vi "Data.OnCompile.Execute.vi"(8 "error in":errorcluster, 10 "VS Ref Groups":T2(array[cluster]) {"VS Refs" format="%.0x"}, 11 "Custom Device Ref":T1 format="%.0x") -> (0 "error out":errorcluster, 3 "Custom Device Ref":T1 format="%.0x")   [LabVIEW 2023, in "Data Access System Explorer.lvlib"]
uses:
  Data Access System Explorer.lvlib
  <vilib>/NI VeriStand/Custom Device API/Custom Device API.lvlib
  <vilib>/NI VeriStand/Custom Device API/Data Reference.ctl
  <vilib>/NI VeriStand/Custom Device API/Block Data Reference.ctl
  <vilib>/NI VeriStand/Custom Device API/Set Item Property (Variant).vi
  <vilib>/NI VeriStand/Custom Device API/Data Access Type.ctl
  <vilib>/NI VeriStand/Custom Device API/Custom Device Item Ref.ctl
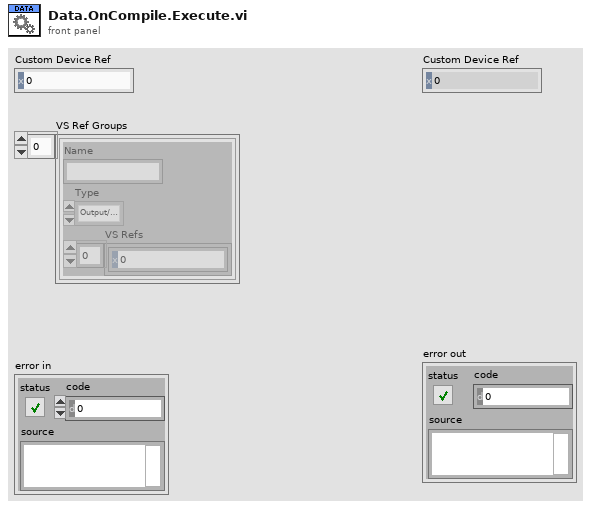
[diagram p1: front panel]
types:
  T1 = typedef "Custom Device API.lvlib/Custom Device Item Ref.ctl" = u64
  T2 = cluster{"Name":string, "Type":enum16{"Output/Write", "Input/Read", "Input/ReadWrite"}, "VS Refs":T1[]}[]
  T3 = typedef "Custom Device API.lvlib/Block Data Reference.ctl" = cluster{"Data Reference":T4, "Offset":u64, "Length":u64}
  T4 = typedef "Custom Device API.lvlib/Data Reference.ctl" = i32
  T5 = cluster{"Refs":T4[], "Values":dbl[], "Reset Values":dbl[]}[]
  T6 = cluster{"Read":cluster{"Refs":T3[], "Values":dbl[]}[], "Write":cluster{"Refs":T3[], "Values":dbl[]}[], "ReadWrite":cluster{"Refs":T4[], "Values":dbl[], "Reset Values":dbl[]}[], "LUT":variant}
  T7 = typedef "Custom Device API.lvlib/Data Access Type.ctl" = enum16{"Read", "Write"}
  T8 = cluster{"Refs":T4[], "Values":dbl[], "Reset Values":dbl[]}
  T9 = enum16{"Output/Write", "Input/Read", "Input/ReadWrite"}
  T10 = typedef "Custom Device API.lvlib/Custom Device Channel.ctl" = cluster{"Type":T11, "Units":string, "Default Value":dbl, "Faultable":bool, "Scalable":bool}
  T11 = typedef "Custom Device API.lvlib/Custom Device Channel Type.ctl" = enum16{"Input", "Output"}
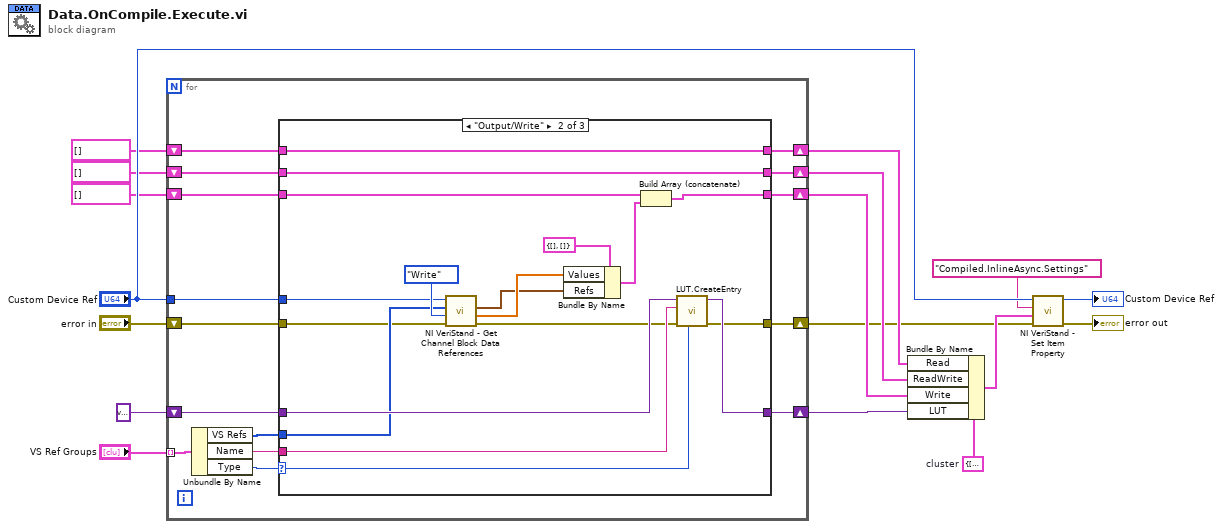
[diagram p0: block diagram]
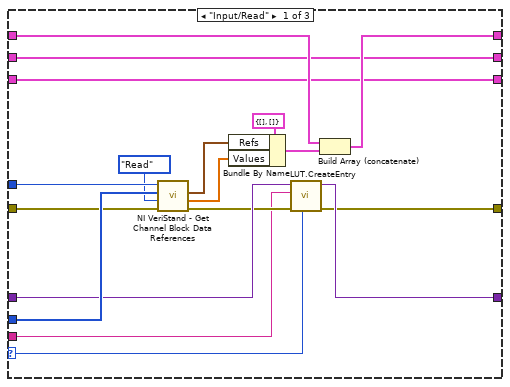
[diagram p2: hidden frame]
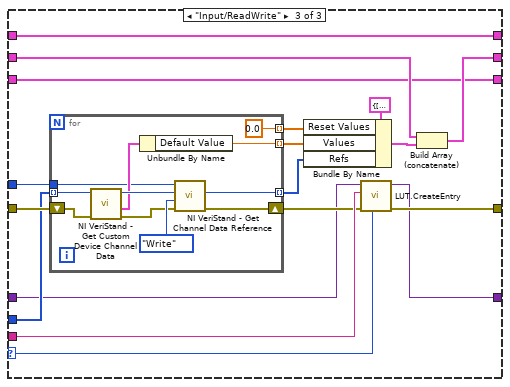
[diagram p3: hidden frame]
diagram:
  w13 = T6 {"Read"=[], "Write"=[], "ReadWrite"=[], "LUT"=variant}  # cluster
  n1 = for {
    tunnel: "VS Ref Groups" -> [w32] mode=indexing
    shift-right: [w30] -> w1
    shift-left: "error in" -> [w31]
    tunnel: "Custom Device Ref" -> [w28]
    shift-right: [w26] -> w2
    shift-left: variant ("LUT") -> [w27]
    shift-right: [w25] -> w4
    shift-left: cluster{"Refs":T3[], "Values":dbl[]}[] [] -> [w20]
    shift-right: [w22] -> w3
    shift-left: T5 [] -> [w21]
    shift-right: [w19] -> w5
    shift-left: cluster{"Refs":T3[], "Values":dbl[]}[] [] -> [w18]
    n2 = Unbundle By Name(w32) -> ("VS Refs"=w29:T1[], "Name"=w24:string, "Type"=w23:T9)
    n3 = case shown="\"Output/Write\"" w23 {
      selector: w23 -> [w38 w64 w79]
      tunnel: w31 -> [w47 w54 w83]
      tunnel: [w45 w65 w77] -> w30
      tunnel: w29 -> [w50 w56 w81]
      tunnel: w28 -> [w49 w57 w74]
      tunnel: w27 -> [w48 w67 w76]
      tunnel: [w46 w66 w75] -> w26
      tunnel: [w35 w62 w69] -> w25
      tunnel: w24 -> [w39 w68 w80]
      tunnel: [w34 w63 w71] -> w22
      tunnel: w21 -> [w34 w63 w73]
      tunnel: w20 -> [w37 w62 w69]
      tunnel: [w33 w60 w70] -> w19
      tunnel: w18 -> [w33 w59 w70]
      frame "Input/Read" {
        n4 = call <vilib>:"NI VeriStand - Get Channel Block Data References.vi"("error in (no error)"=w47, "Access"=Data_Access_Type."Read", "Channel Refs"=w50, "Device Ref in"=w49) -> ("error out"=w41:errorcluster, "Values Array"=w42:dbl[], "Block Data Refs"=w43:T3[])  [unwired: 4 in, 1 out]
        n5 = Bundle By Name(cluster=cluster{"Refs":T3[], "Values":dbl[]} {"Refs"=[], "Values"=[]}, "Refs"=w43, "Values"=w42) -> (w36:cluster{"Refs":T3[], "Values":dbl[]})
        n6 = call "LUT.CreateEntry.vi"("Type"=w38, "error in (no error)"=w41, "Name"=w39, "LUT"=w48) -> ("error out"=w45:errorcluster, "LUT"=w46:variant)  [unwired: 6 in]
        n7 = Build Array (concatenate)(w37, w36) -> (w35:cluster{"Refs":T3[], "Values":dbl[]}[])
      }
      frame "Output/Write" {
        n8 = call <vilib>:"NI VeriStand - Get Channel Block Data References.vi"("error in (no error)"=w54, "Access"=Data_Access_Type."Write", "Channel Refs"=w56, "Device Ref in"=w57) -> ("error out"=w53:errorcluster, "Values Array"=w55:dbl[], "Block Data Refs"=w51:T3[])  [unwired: 4 in, 1 out]
        n9 = Bundle By Name(cluster=cluster{"Refs":T3[], "Values":dbl[]} {"Refs"=[], "Values"=[]}, "Values"=w55, "Refs"=w51) -> (w61:cluster{"Refs":T3[], "Values":dbl[]})
        n10 = Build Array (concatenate)(w59, w61) -> (w60:cluster{"Refs":T3[], "Values":dbl[]}[])
        n11 = call "LUT.CreateEntry.vi"("Type"=w64, "error in (no error)"=w53, "Name"=w68, "LUT"=w67) -> ("error out"=w65:errorcluster, "LUT"=w66:variant)  [unwired: 6 in]
      }
      frame "Input/ReadWrite" {
        n12 = for {
          shift-right: [w96] -> w78
          shift-left: w83 -> [w94]
          tunnel: [w91] -> w86 mode=indexing
          tunnel: [w90] -> w85 mode=indexing
          tunnel: [0.0] -> w84 mode=indexing
          tunnel: w81 -> [w88] mode=indexing
          tunnel: w74 -> [w87]
          n13 = call <vilib>:"NI VeriStand - Get Custom Device Channel Data.vi"("error in (no error)"=w94, "Channel Ref in"=w88) -> ("error out"=w93:errorcluster, "Channel"=w92:T10, "Channel Ref out"=w95:T1)  [unwired: 4 in, 3 out]
          n14 = Unbundle By Name(w92) -> ("Default Value"=w91:dbl)
          n15 = call <vilib>:"NI VeriStand - Get Channel Data Reference.vi"("error in (no error)"=w93, "Access"=Data_Access_Type."Write", "Channel Ref in"=w95, "Device Ref in"=w87) -> ("error out"=w96:errorcluster, "Channel Data Reference"=w90:T4)  [unwired: 5 in, 1 out]
        }
        n16 = Bundle By Name(cluster=T8 {"Refs"=[], "Values"=[], "Reset Values"=[]}, "Reset Values"=w84, "Values"=w86, "Refs"=w85) -> (w72:T8)
        n17 = call "LUT.CreateEntry.vi"("Type"=w79, "error in (no error)"=w78, "Name"=w80, "LUT"=w76) -> ("error out"=w77:errorcluster, "LUT"=w75:variant)  [unwired: 6 in]
        n18 = Build Array (concatenate)(w73, w72) -> (w71:T5)
      }
    }
  }
  n19 = Bundle By Name(cluster=w13, "Read"=w4, "ReadWrite"=w3, "Write"=w5, "LUT"=w2) -> (w14:T6)
  n20 = call-poly <vilib>:"NI VeriStand - Set Item Property.vi"("error in (no error)"=w1, "Value"=w14, "Property Name"="Compiled.InlineAsync.Settings", "Item Ref in"="Custom Device Ref") -> ("error out"=→"error out":errorcluster, "Item Ref out"=→"Custom Device Ref":T1)  [unwired: 5 in, 1 out]
